vi "GetCommand _OC Trim_.vi"(0 "object in":refnum<class "WK6425.lvclass">, 5 "error in (no error)":errorcluster) -> (14 "object out":refnum<class "WK6425.lvclass">, 15 "Command _OC Trim_":string, 19 "error out":errorcluster)   [LabVIEW 2013, in "WK6425.lvclass"]
uses:
  WK6425.lvclass
  WK6425.lvclass/WK6425.ctl
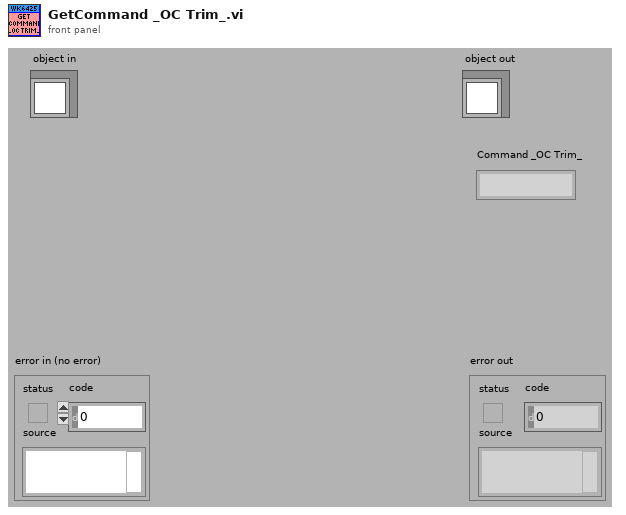
[diagram p1: front panel]
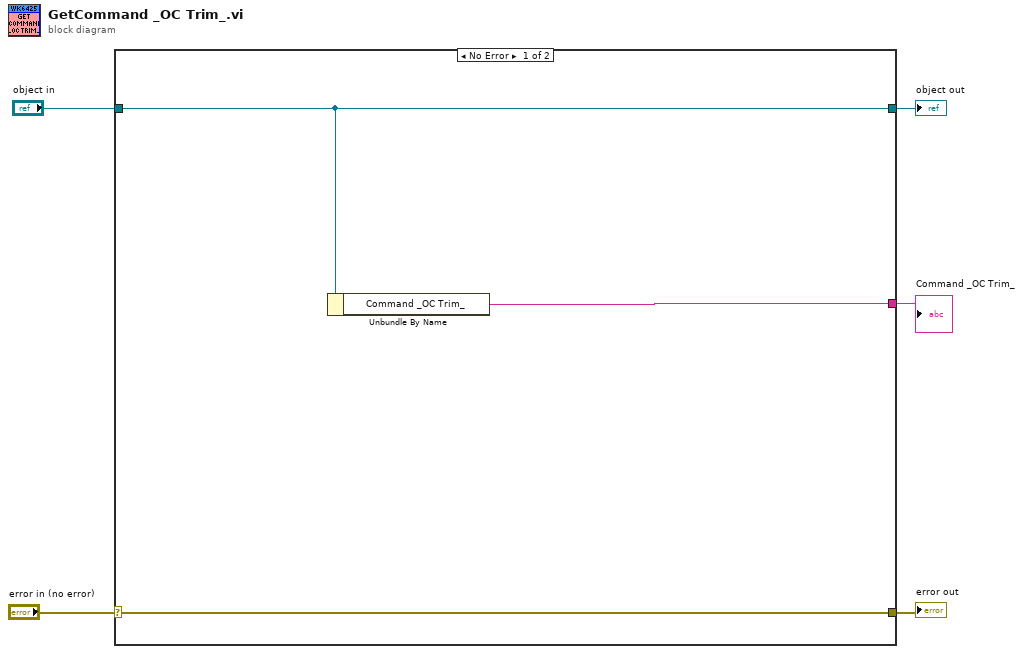
[diagram p0: block diagram]
diagram:
  n1 = case shown="No Error" "error in (no error)" {
    selector: "error in (no error)" -> [w7 w10]
    tunnel: [w7 w10] -> w4
    tunnel: [w6 w9] -> w2
    tunnel: "object in" -> [w6 w9]
    tunnel: [w8 _] -> w1
    frame No Error {
      n2 = Unbundle By Name(w6) -> ("Command _OC Trim_"=w8:string)
    }
    frame Error {
    }
  }
  "error out" <- w4
  "object out" <- w2
  "Command _OC Trim_" <- w1
